vi "NI_FPGA_PPG.get status.vi"(0 "i ref in":refnum<vi>, 3 "ms timeout (10000)":i32=10000, 5 "error in (no error)":errorcluster) -> (14 "i ref out":refnum<vi>, 16 "FPGA_status":i32, 17 "timed out":bool, 19 "error out":errorcluster)   [LabVIEW 2014, in "NI_FPGA_PPG.lvlib"]
doc: "Queries the execution status of the FPGA (Idle = 0, Running = 4).\n\nLicense Agreement for this software:\n\nCopyright (C) 2009\nFalk Ziegler\nInstitut für Physik\nErnst-Moritz-Arndt Universität\nFelix-Hausdorff-Str. 6\n17487 Greifswald\n\nContact: Falk Ziegler, ziegler@physik.uni-greifswald.de\n\nThis program is free software: you can redistribute it and/or modify it under the terms of the GNU General Public License as published by the Free Software Foundation, either version 3 of the License, or (at your option) any later version.\n\nThis program is distributed in the hope that it will be useful, but WITHOUT ANY WARRANTY; without even the implied warranty of MERCHANTABILITY or FITNESS FOR A PARTICULAR PURPOSE. See the GNU General Public License for more details.\n\nYou should have received a copy of the GNU General Public License along with this program. If not, see <http://www.gnu.org/licenses/>.\n\nFor all questions and ideas contact: ziegler@physik.uni-greifswald.de or d.beck@gsi.de\nLast update: 01-Sep-2009"
uses:
  NI_FPGA_PPG.lvlib
  CSCore/CSApplicationBaseClasses/DeviceBase/DeviceBase.lvlib
  CSinstr.lib/NI_FPGA_PPG/host/instrumentDriver/NI-FPGA_PPG_Driver.lvlib
  CSlibraries/UtilityLib/UtilityLib.lvlib
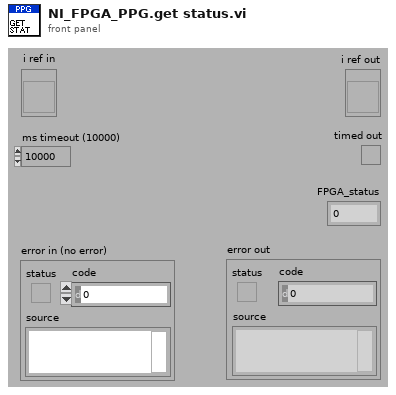
[diagram p1: front panel]
types:
  T1 = typedef "NI_FPGA_PPG.lvlib/NI_FPGA_PPG.i attribute.ctl" = cluster{"dim_service_id":cluster{"dim_actual_device_status":i32, "dim_event_data":i32, "dim_cmd_data":i32, "dim_cmd_data _description":i32, "dim_channel_description":i32}, "VISA":refnum<visa-resource-name>, "actual_device_status":i32, "event_data_id":i32, "pdc_enabled":bool, "pdc_timestamp":u32, "cmd_data_string":string, "cmd_data_size":i32, "cmd_data_description_string":string, "cmd_data_description_size":i32, "channel_description_string":string, "channel_description_size":i32}
  T2 = typedef "NI-FPGA_PPG_Driver.lvlib/FPGA_target_state_type.ctl" = enum16{"idle", "reset", "query", "load", "run", "stopped"}
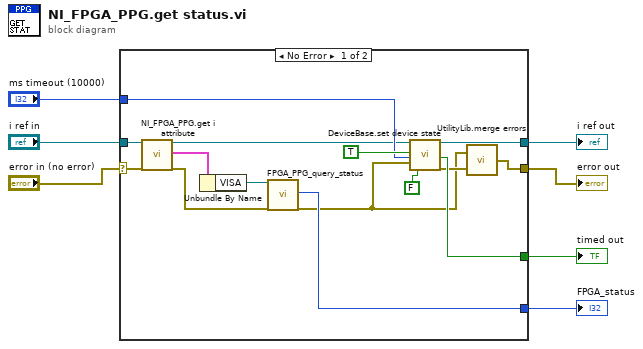
[diagram p0: block diagram]
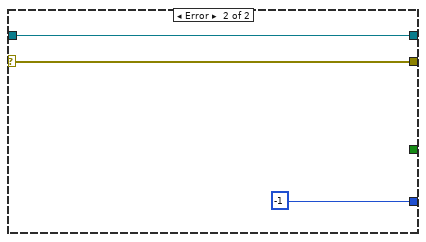
[diagram p2: hidden frame]
diagram:
  n1 = case shown="No Error" "error in (no error)" {
    selector: "error in (no error)" -> [w21 w24]
    tunnel: "i ref in" -> [w22 w25]
    tunnel: [w17 w25] -> w5
    tunnel: [w10 w24] -> w4
    tunnel: "ms timeout (10000)" -> [w14 _]
    tunnel: [w12 _] -> w2
    tunnel: [w11 -1] -> w1
    frame No Error {
      n2 = call "NI_FPGA_PPG.get i attribute.vi"("i ref in"=w22, "error in (no error)"=w21) -> ("i ref out"=w13:refnum<vi>, "i attribute"=w20:T1, "error out"=w18:errorcluster)  [unwired: 15 in]
      n3 = Unbundle By Name(w20) -> ("VISA"=w19:refnum<visa-resource-name>)
      n4 = call "FPGA_PPG_query_status.vi"("resource_in"=w19, "error in (no error)"=w18) -> ("FPGA_state"=w11:T2, "error out"=w8:errorcluster)  [unwired: 15 in, 1 out]
      n5 = call "DeviceBase.set device state.vi"("i ref in"=w13, "implicit"=TRUE, "ms timeout (10000)"=w14, "device error"=w8, "mayResetError (FALSE)"=FALSE) -> ("i ref out"=w17:refnum<vi>, "timed out"=w12:bool, "error out"=w9:errorcluster)  [unwired: 12 in]
      n6 = call "UtilityLib.merge errors.vi"("error2 (no error)"=w9, "error1 (no error)"=w8) -> ("error out"=w10:errorcluster)
    }
    frame Error {
    }
  }
  "error out" <- w4
  "i ref out" <- w5
  "timed out" <- w2
  "FPGA_status" <- w1
